vi "Fundamental-Nonfundamental Powers Calculation.vi"() -> ()   [LabVIEW 2021]
uses:
  Typedefs/Fundamental Powers Values.ctl
  Typedefs/Nonfundamental Powers Values.ctl
  <vilib>/measure/matone.llb/Extract Single Tone Information 1 Chan.vi
  <vilib>/measure/NI_MAPro.lvlib
  <vilib>/ptbypt/NI_PtbyPt.lvlib
panel:
  out "Nonfundamental Powers Values":T1
  out "Fundamental Powers Values":T2
  out "Error Out":errorcluster
  in  "Error In":errorcluster
  in  "Current Waveform":waveform(dbl)
  in  "Voltage Waveform":waveform(dbl)
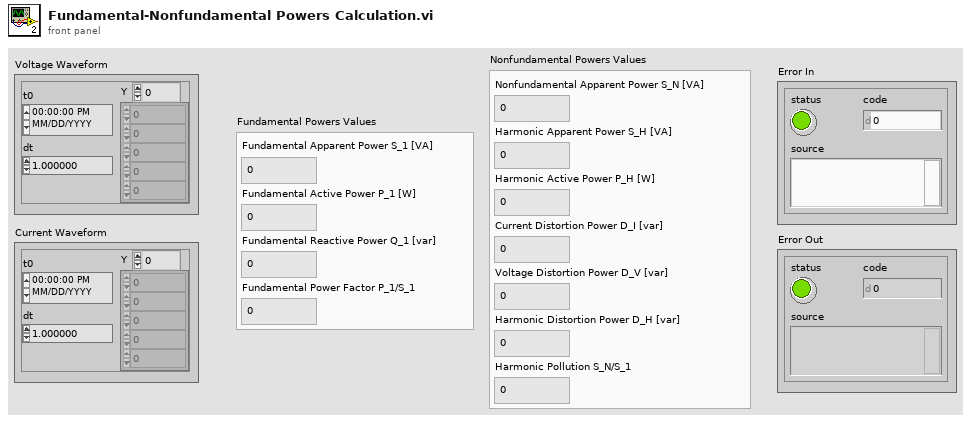
[diagram p1: front panel]
types:
  T1 = typedef "Nonfundamental Powers Values.ctl" = cluster{"Nonfundamental Apparent Power S_N [VA]":dbl, "Harmonic Apparent Power S_H [VA]":dbl, "Harmonic Active Power P_H [W]":dbl, "Current Distortion Power D_I [var]":dbl, "Voltage Distortion Power D_V [var]":dbl, "Harmonic Distortion Power D_H [var]":dbl, "Harmonic Pollution S_N/S_1":dbl}
  T2 = typedef "Fundamental Powers Values.ctl" = cluster{"Fundamental Apparent Power S_1 [VA]":dbl, "Fundamental Active Power P_1 [W]":dbl, "Fundamental Reactive Power Q_1 [var]":dbl, "Fundamental Power Factor P_1/S_1":dbl}
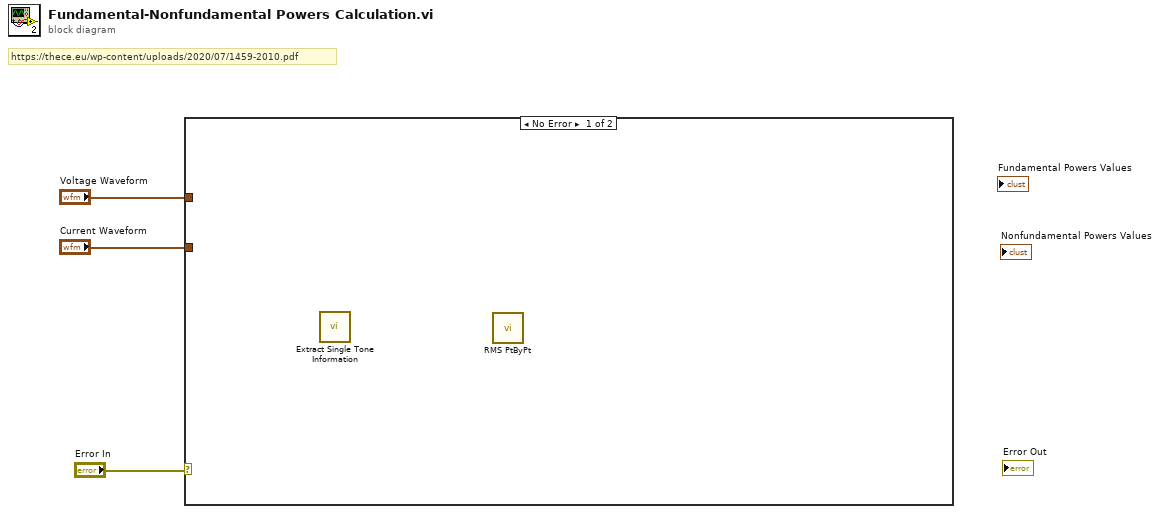
[diagram p0: block diagram]
diagram:
  # "https://thece.eu/wp-content/uploads/2020/07/1459-2010.pdf"
  n1 = case shown="No Error" "Error In" {
    tunnel: "Voltage Waveform" -> [_ _]
    tunnel: "Current Waveform" -> [_ _]
    frame No Error {
      n2 = call-poly <vilib>:"Extract Single Tone Information.vi"() -> ()  [unwired: 6 in, 6 out]
      n3 = call <vilib>:"RMS PtByPt.vi"() -> ()  [unwired: 4 in, 2 out]
    }
    frame Error {
    }
  }
